vi "Main.vi"() -> ()   [LabVIEW 2017, in "Chain of Responsibility Pattern Demo.lvclass"]
uses:
  Chain of Responsibility Pattern Demo.lvclass
  Add Class/Add.lvclass
  Subtract Class/Subtract.lvclass
  C:/Users/fflores/Documents/LabVIEW-Open-Projects/LabIVEW OOP Design Patterns/Chain of Responsibility Pattern/Chain Class/Chain.lvclass
  Multiply Class/Multiply.lvclass
  Divide Class/Divide.lvclass
  Numbers Class/Numbers.lvclass
  ConsoleOut/Print Options.ctl
panel:
  in  "CalculationWanted":string="Add"
  in  "Number2":dbl=5.0
  in  "Number1":dbl=10.0
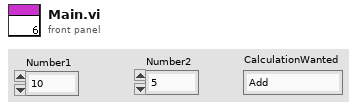
[diagram p1: front panel]
types:
  T1 = typedef "Print Options.ctl" = enum16{"Create", "Get Reference", "Print", "Print Header", "Close"}
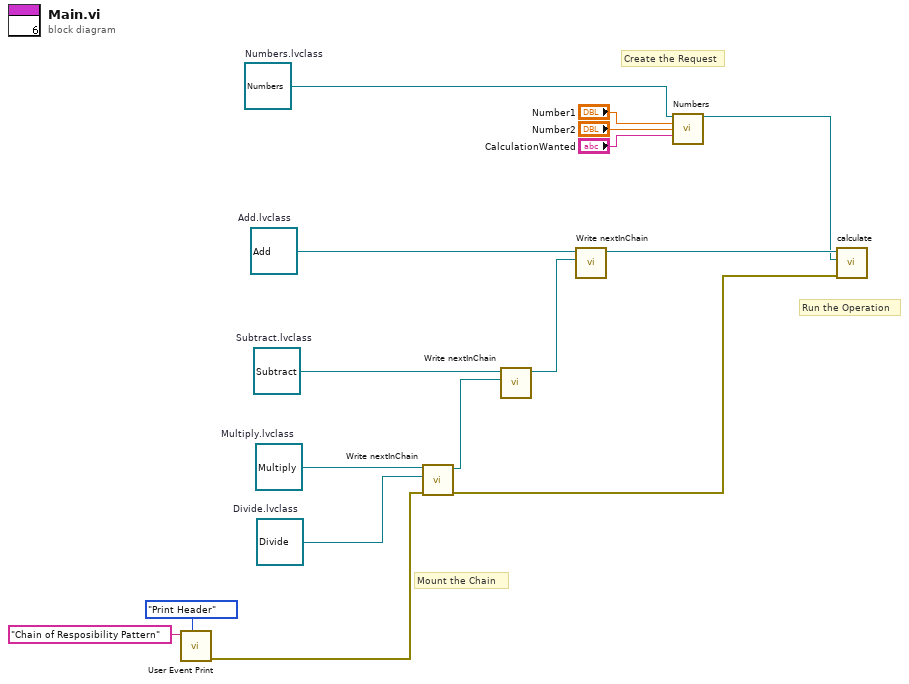
[diagram p0: block diagram]
diagram:
  w7 = refnum<class "Numbers.lvclass"> refnum  # Numbers.lvclass
  w13 = refnum<class "Divide.lvclass"> refnum  # Divide.lvclass
  w14 = refnum<class "Multiply.lvclass"> refnum  # Multiply.lvclass
  w15 = refnum<class "Subtract.lvclass"> refnum  # Subtract.lvclass
  w16 = refnum<class "Add.lvclass"> refnum  # Add.lvclass
  # "Run the Operation"
  # "Create the Request"
  # "Mount the Chain"
  n1 = call "User Event Print.vi"("Options"=Print_Options."Print Header", "String to Print"="Chain of Resposibility Pattern") -> ("error out"=w3:errorcluster)  [unwired: 8 in, 1 out]
  n2 = call-dynamic "Write nextInChain.vi"("error in (no error)"=w3, "Chain.lvclass"=w13, "Multiply in"=w14) -> ("error out"=w6:errorcluster, "Multiply out"=w5:refnum<class "Multiply.lvclass">)  [unwired: 7 in]
  n3 = call-dynamic "Write nextInChain.vi"("Chain.lvclass"=w5, "Subtract in"=w15) -> ("Subtract out"=w4:refnum<class "Subtract.lvclass">)  [unwired: 8 in, 1 out]
  n4 = call-dynamic "Write nextInChain.vi"("Chain.lvclass"=w4, "Add in"=w16) -> ("Add out"=w9:refnum<class "Add.lvclass">)  [unwired: 8 in, 1 out]
  n5 = call "Numbers.vi"("Numbers in"=w7, "Number1"="Number1", "Number2"="Number2", "CalculationWanted"="CalculationWanted") -> ("Numbers out"=w8:refnum<class "Numbers.lvclass">)  [unwired: 10 in, 1 out]
  n6 = call-dynamic "calculate.vi"("error in (no error)"=w6, "Numbers.lvclass"=w8, "Add in"=w9) -> ()  [unwired: 7 in, 2 out]
